vi "Create.vi"(8 "error in (no error)":errorcluster, 10 "Tolerance":dbl) -> (0 "error out":errorcluster, 3 "Tolerant Numeric Comparator Out":refnum<class "Tolerant Numeric Input Comparator.lvclass">)   [LabVIEW 2020, in "Tolerant Numeric Input Comparator.lvclass"]
uses:
  Tolerant Numeric Input Comparator.lvclass
  Tolerant Numeric Input Comparator.lvclass/Tolerant Numeric Input Comparator.ctl
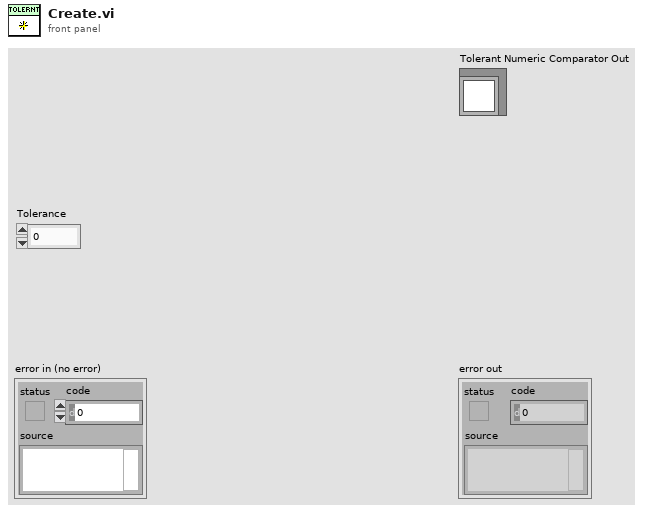
[diagram p1: front panel]
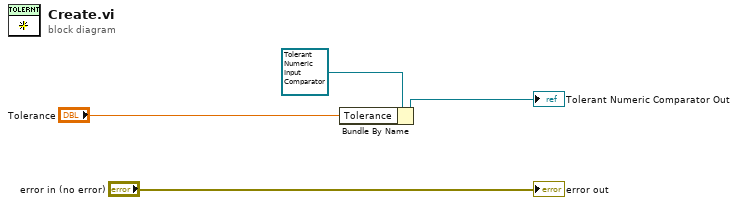
[diagram p0: block diagram]
diagram:
  n1 = Bundle By Name(cluster=refnum<class "Tolerant Numeric Input Comparator.lvclass"> refnum ("Tolerant Numeric Comparator"), "Tolerance"="Tolerance") -> (→"Tolerant Numeric Comparator Out":refnum<class "Tolerant Numeric Input Comparator.lvclass">)
  "error out" <- "error in (no error)"
